vi "execute.vi"(7 "first call?":bool, 8 "error in (no error)":errorcluster, 9 "result allocation":T1, 10 "parameters":T1, 11 "action in":refnum<class "action.lvclass">) -> (0 "error out":errorcluster, 1 "results":T1, 2 "parameter allocation":T1, 3 "action out":refnum<class "action.lvclass">, 4 "complete?":bool)   [LabVIEW 2014, in "action.lvclass"]
doc: "Provides an interface for other Action implementations to use. Requires calling code to provide 'First Call?' so that implementations can be non-blocking and called repeatedly. Once finished, the implementation should return 'complete?' as True."
uses:
  action.lvclass
  <vilib>/NI/Tag Bus/table/data table.ctl
  <vilib>/NI/Tag Bus/table/data table.lvlib
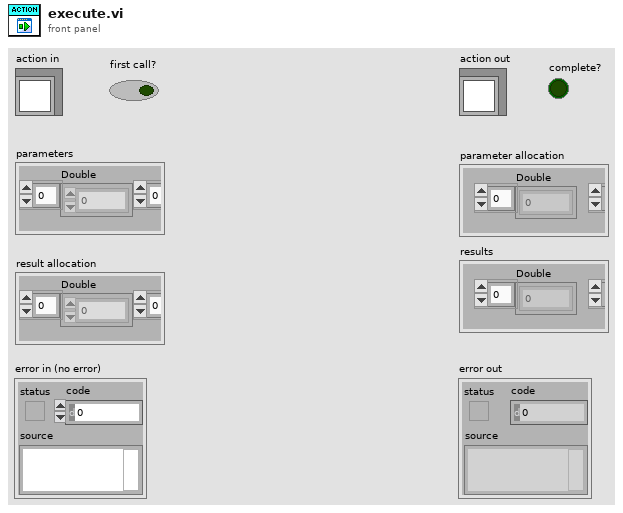
[diagram p1: front panel]
types:
  T1 = typedef "tag bus.lvlib/data table.lvlib/data table.ctl" = cluster{"Double":dbl[], "Single":sgl[], "I64":i64[], "I32":i32[], "I16":i16[], "I8":i8[], "U64":u64[], "U32":u32[], "U16":u16[], "U8":u8[], "Boolean":bool[], "String":string[], "Array of Double":cluster{"DBL Array":dbl[]}[], "Array of Single":cluster{"SGL Array":sgl[]}[], "Array of I64":cluster{"I64 Array":i64[]}[], "Array of I32":cluster{"I32 Array":i32[]}[], "Array of I16":cluster{"I16 Array":i16[]}[], "Array of I8":cluster{"I8 Array":i8[]}[], "Array of U64":cluster{"U64 Array":u64[]}[], "Array of U32":cluster{"U32 Array":u32[]}[], "Array of U16":cluster{"U16 Array":u16[]}[], "Array of U8":cluster{"U8 Array":u8[]}[], "Array of Boolean":cluster{"Boolean Array":bool[]}[], "Array of String":cluster{"String Array":string[]}[]}
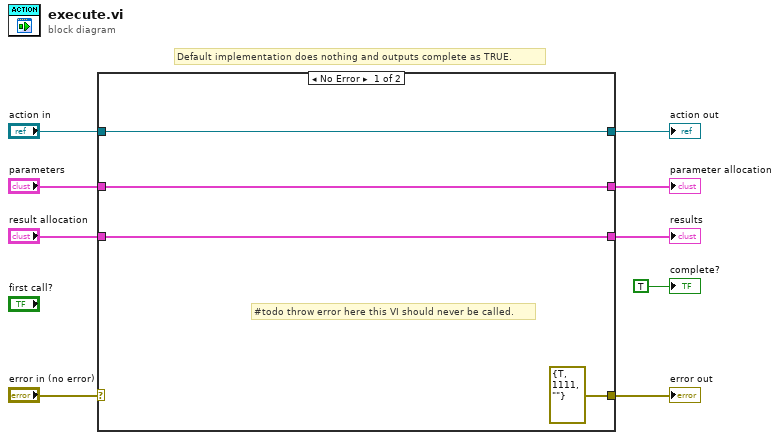
[diagram p0: block diagram]
diagram:
  # "Default implementation does nothing and outputs complete as TRUE."
  n1 = case shown="No Error" "error in (no error)" {
    selector: "error in (no error)" -> [_ w17]
    tunnel: [errorcluster {"status"=TRUE, "code"=1111, "source"=""} ("error IO") w17] -> w8
    tunnel: [w13 w16] -> w6
    tunnel: "action in" -> [w13 w16]
    tunnel: [w12 w15] -> w5
    tunnel: "parameters" -> [w12 w15]
    tunnel: "result allocation" -> [w11 w14]
    tunnel: [w11 w14] -> w2
    frame No Error {
      # "#todo throw error here this VI should never be called."
    }
    frame Error {
    }
  }
  "error out" <- w8
  "action out" <- w6
  "parameter allocation" <- w5
  "results" <- w2
  "complete?" <- TRUE ("complete?")
